vi "Fit Parameters.vi"(8 "error in":errorcluster, 10 "PAS Cell Data in":refnum<class "PAS Cell Data.lvclass">=refnum, 11 "PAS File Obs in":refnum<class "PAS File Obs.lvclass">) -> (0 "error out":errorcluster, 2 "PAS Cell Data Out":refnum<class "PAS Cell Data.lvclass">, 3 "PAS File Obs Out":refnum<class "PAS File Obs.lvclass">)   [LabVIEW 2014, in "PAS File Obs.lvclass"]
uses:
  PAS File Obs.lvclass
  Main/Controls/Cell Data.ctl
  <vilib>/Analysis/Matrix/NI_Matrix.lvlib
  <vilib>/Analysis/Matrix/Numeric/Conversions/Matrix To Array - RM.vi
  Data/Cell/PAS Cell Data.lvclass
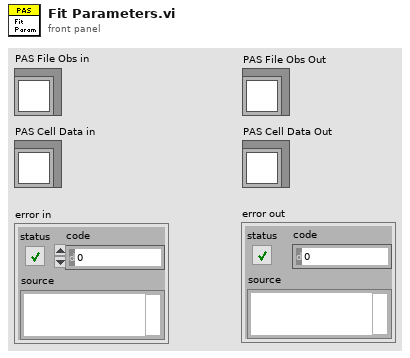
[diagram p1: front panel]
types:
  T1 = enum16{"big-endian, network order", "native, host order", "little-endian"}
  T2 = typedef "Cell Data.ctl" = u8
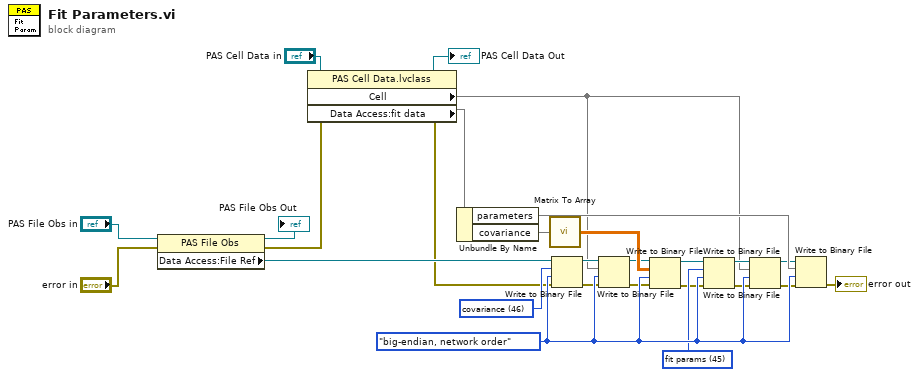
[diagram p0: block diagram]
diagram:
  w25 = T1."big-endian, network order" ("byte order (0:big-endian, network order)")
  w21 = T2 45 items=["TEC SP"=23, "TEC Enable"=24, "Qsp"=25, "Tac"=26, "Pac"=27, "Q0ac"=28, "Qac"=29, "Cell TEC T (T1)"=30, "Tmain"=31, "Tv"=32, "RHv"=33, "lasRMS"=34, "dPhi"=35, "Tau"=36, "Cell Q"=37, "f0"=38, "Integrated Area"=39, "Max Amplitude"=40, "Noise Limit"=41, "Lower Noise Bound"=42, "Upper Noise Bound"=43, "Absorption"=44, "fit params"=45, "covariance"=46] ("cellNumData")
  w11 = T2 46 items=["TEC SP"=23, "TEC Enable"=24, "Qsp"=25, "Tac"=26, "Pac"=27, "Q0ac"=28, "Qac"=29, "Cell TEC T (T1)"=30, "Tmain"=31, "Tv"=32, "RHv"=33, "lasRMS"=34, "dPhi"=35, "Tau"=36, "Cell Q"=37, "f0"=38, "Integrated Area"=39, "Max Amplitude"=40, "Noise Limit"=41, "Lower Noise Bound"=42, "Upper Noise Bound"=43, "Absorption"=44, "fit params"=45, "covariance"=46] ("cellNumData")
  n1 = property class="PAS File Obs"(reference="PAS File Obs in", error in="error in") -> (reference out=→"PAS File Obs Out":refnum<class "PAS File Obs.lvclass">, error out=w3:errorcluster, "Data Access:File Ref"=w6:refnum<file>)
  n2 = property class="PAS Cell Data.lvclass"(reference="PAS Cell Data in", error in=w3) -> (reference out=→"PAS Cell Data Out":refnum<class "PAS Cell Data.lvclass">, error out=w2:errorcluster, "Cell"=w9, "Data Access:fit data"=w8)
  n3 = Unbundle By Name(w8) -> ("parameters"=w26, "covariance"=w27)
  n4 = call-poly <vilib>:"Matrix To Array.vi"("Real Matrix"=w27) -> ("Real 2D Array"=w20:dbl[][])
  n5 = Write to Binary File(file (use dialog)=w6, data=w11, error in=w2, 9:w25) -> (refnum out=w13:refnum<file>, error out=w12:errorcluster)  [unwired: 2 in, 1 out]
  n6 = Write to Binary File(file (use dialog)=w13, data=w9, error in=w12, 9:w25) -> (refnum out=w14:refnum<file>, error out=w15:errorcluster)  [unwired: 2 in, 1 out]
  n7 = Write to Binary File(file (use dialog)=w14, data=w20, error in=w15, 9:w25) -> (refnum out=w16:refnum<file>, error out=w17:errorcluster)  [unwired: 2 in, 1 out]
  n8 = Write to Binary File(file (use dialog)=w16, data=w21, error in=w17, 9:w25) -> (refnum out=w18:refnum<file>, error out=w19:errorcluster)  [unwired: 2 in, 1 out]
  n9 = Write to Binary File(file (use dialog)=w18, data=w9, error in=w19, 9:w25) -> (refnum out=w22:refnum<file>, error out=w23:errorcluster)  [unwired: 2 in, 1 out]
  n10 = Write to Binary File(file (use dialog)=w22, data=w26, error in=w23, 9:w25) -> (error out=→"error out":errorcluster)  [unwired: 2 in, 2 out]
